vi "matrici_v0_v43.vi"() -> ()   [LabVIEW 2009]
uses:
  <vilib>/Native 3D Graph/xcontrol/3DPC_SurfacePlot.xctl
  <vilib>/Native 3D Graph/classes/Line/Line.lvclass
panel:
  in  "stop":bool
  out "3D Graph":refnum<class "Base Datatype.lvclass">[](xcontrol)
  out "X":dbl=3.326794657762937
  in  "Domeniul de definitie x":dbl(slide)=6.653589315525876 scale=0.5..10.0
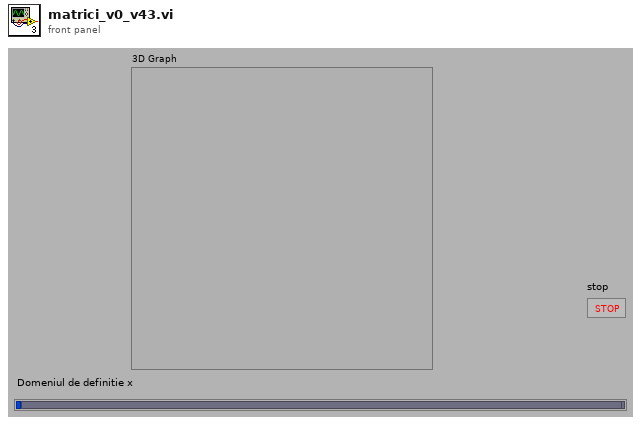
[diagram p1: front panel]
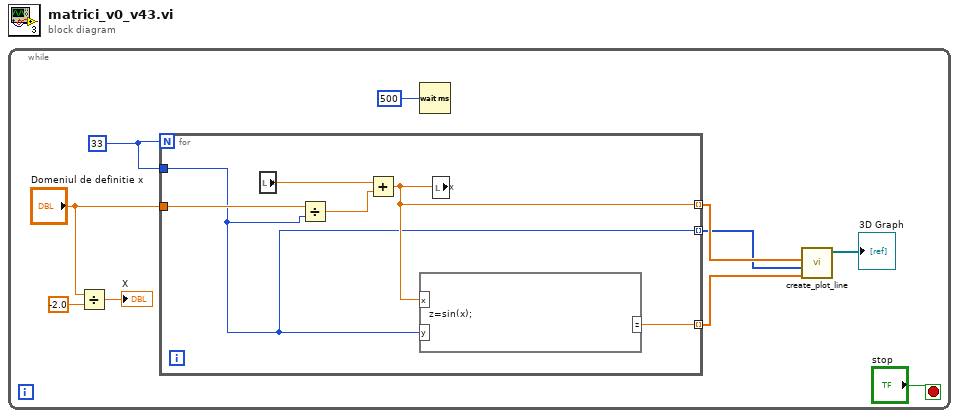
[diagram p0: block diagram]
diagram:
  n1 = while {
    stop <- "stop" stop-if-true
    w9 = 33
    n2 = Divide(x="Domeniul de definitie x", y=-2.0) -> (x/y=→"X":dbl)
    n3 = for {
      N: w9 -> [_]
      tunnel: [w13] -> w5 mode=indexing
      tunnel: w9 -> [w11]
      tunnel: "Domeniul de definitie x" -> [w15]
      tunnel: [w12] -> w3 mode=indexing
      tunnel: [w11] -> w4 mode=indexing
      n4 = local read "X"() -> (w16:dbl)
      n5 = Divide(x=w15, y=w11) -> (x/y=w14:dbl)
      n6 = Add(x=w16, y=w14) -> (x+y=w13:dbl)
      n7 = formula code="z=sin(x);"("x"=w13, "y"=w11) -> ("z"=w12:dbl)
      n8 = local write "X"(w13) -> ()
    }
    n9 = Wait (ms)(milliseconds to wait=500) -> ()  [unwired: 1 out]
    n10 = call <vilib>:"create_plot_line.vi"("z vector"=w3, "y vector"=w4, "x vector"=w5) -> ("plots out"=→"3D Graph":refnum<class "Base Datatype.lvclass">[])  [unwired: 2 in, 6 out]
  }
